vi "Handle Event.vi"(8 "error in (no error)":errorcluster, 9 "Controller in":refnum<class "Controller.lvclass">, 10 "Event Data":refnum<class "Event.lvclass">, 11 "Update Boolean Msg in":refnum<class "Update Boolean Event Msg.lvclass">) -> (0 "error out":errorcluster, 1 "Controller out":refnum<class "Controller.lvclass">, 3 "Update Boolean Msg out":refnum<class "Update Boolean Event Msg.lvclass">)   [LabVIEW 2023, in "Example MVC Actors.lvlib" / "Example Controller.lvlib" / "Update Boolean Event Msg.lvclass"]
uses:
  Update Boolean Event Msg.lvclass
  Event/Event.lvclass
  Controller/Controller.lvclass
  Example Controller/Example Controller.lvclass
  Example Events/Boolean Event.lvclass
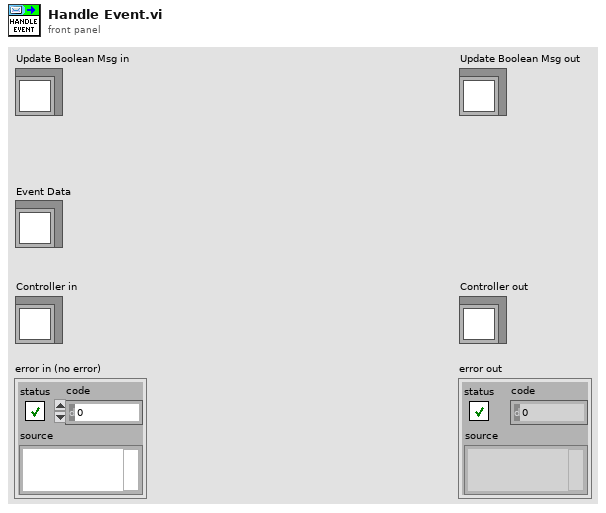
[diagram p1: front panel]
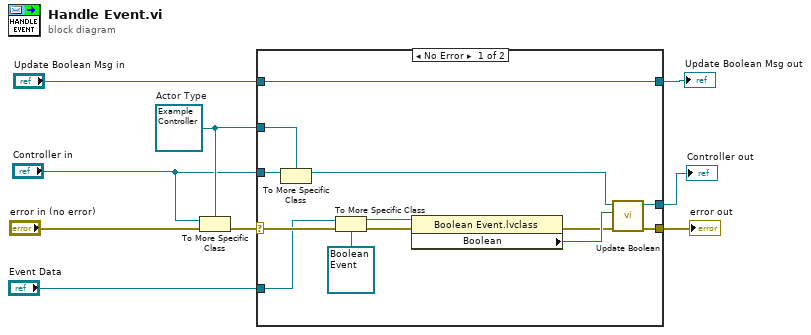
[diagram p0: block diagram]
diagram:
  w8 = refnum<class "Example Controller.lvclass"> refnum  # Actor Type
  n1 = To More Specific Class(target class=w8, reference="Controller in", error in="error in (no error)") -> (error out=w9:errorcluster)  [unwired: 1 out]
  n2 = case shown="No Error" w9 {
    selector: w9 -> [w20 w24]
    tunnel: "Controller in" -> [w17 w25]
    tunnel: "Update Boolean Msg in" -> [w14 w23]
    tunnel: [w21 w24] -> w1
    tunnel: w8 -> [w18 _]
    tunnel: [w16 w25] -> w3
    tunnel: "Event Data" -> [w15 _]
    tunnel: [w14 w23] -> w5
    frame No Error {
      n3 = To More Specific Class(target class=w18, reference=w17) -> (specific class reference=w19:refnum<class "Example Controller.lvclass">)  [unwired: 1 in, 1 out]
      n4 = To More Specific Class(target class=refnum<class "Boolean Event.lvclass"> refnum ("Example Source.lvlib:Boolean Event.lvclass"), reference=w15, error in=w20) -> (specific class reference=w12:refnum<class "Boolean Event.lvclass">, error out=w13:errorcluster)
      n5 = property class="Boolean Event.lvclass"(reference=w12, error in=w13) -> (error out=w10:errorcluster, "Boolean"=w11:bool)  [unwired: 1 out]
      n6 = call "Update Boolean.vi"("error in (no error)"=w10, "Boolean"=w11, "Example Controller in"=w19) -> ("error out"=w21:errorcluster, "Example Controller out"=w16:refnum<class "Example Controller.lvclass">)  [unwired: 7 in]
    }
    frame Error {
    }
  }
  "error out" <- w1
  "Update Boolean Msg out" <- w5
  "Controller out" <- w3
